vi "test-trajectory-generator-ALL.vi"(8 "error in (no error)":errorcluster) -> (0 "error out":errorcluster, 3 "ALL TESTS PASSED":bool)   [LabVIEW 2019]
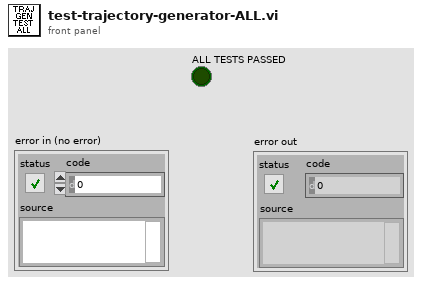
[diagram p1: front panel]
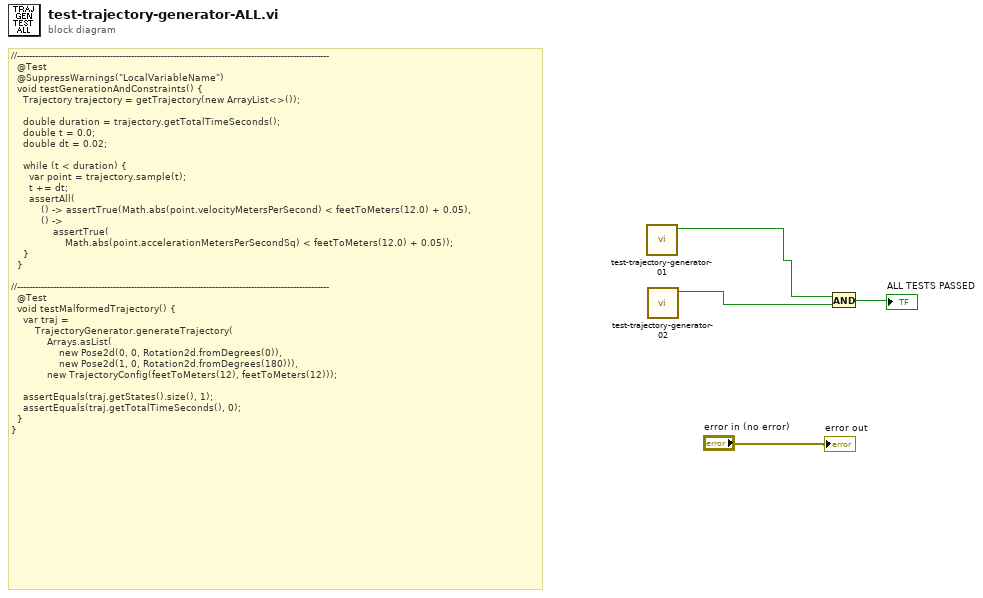
[diagram p0: block diagram]
diagram:
  # "//--------------------------------------------------------------------------------------------------------\n  @Test\n  @SuppressWarnings(\"LocalVariableName\")\n  void testGenerationAndConstraints() {\n    Trajectory trajectory = getTrajectory(new ArrayList<>());\n\n    double duration = trajectory.getTotalTimeSeconds();\n    double t = 0.0;\n    double dt = 0.02;\n\n    while (t < duration) {\n      var point = trajectory.sample(t);\n      t += dt;\n      assertAll(\n          () -> assertTrue(Math.abs(point.velocityMetersPerSecond) < feetToMeters(12.0) + 0.05),\n          () ->\n              assertTrue(\n                  Math.abs(point.accelerationMetersPerSecondSq) < feetToMeters(12.0) + 0.05));\n    }\n  }\n\n//--------------------------------------------------------------------------------------------------------\n  @Test\n  void testMalformedTrajectory() {\n    var traj =\n        TrajectoryGenerator.generateTrajectory(\n            Arrays.asList(\n                new Pose2d(0, 0, Rotation2d.fromDegrees(0)),\n                new Pose2d(1, 0, Rotation2d.fromDegrees(180))),\n            new TrajectoryConfig(feetToMeters(12), feetToMeters(12)));\n\n    assertEquals(traj.getStates().size(), 1);\n    assertEquals(traj.getTotalTimeSeconds(), 0);\n  }\n}"
  n1 = call "test-trajectory-generator-01.vi"() -> ("Okay"=w3:bool)  [unwired: 11 in]
  n2 = call "test-trajectory-generator-02.vi"() -> ("Okay"=w2:bool)  [unwired: 11 in]
  n3 = And(x=w3, y=w2) -> (x .and. y?=→"ALL TESTS PASSED":bool)
  "error out" <- "error in (no error)"
